vi "Modify Test Data.vi"(11 "Field Values in":T1={"cpu_temp"=48.25, "error_code"=-9003, "cpu_load"=8, "cpu_type"="Ryzen 5 2600", "cpu_busy?"=FALSE}) -> (2 "Variant":variant, 3 "Field Values out":T1={"cpu_temp"=48.25, "error_code"=-9003, "cpu_load"=8, "cpu_type"="Ryzen 5 2600", "cpu_busy?"=FALSE})   [LabVIEW 2020, in "InfluxDB v2 Client.lvlib"]
doc: "Modifies the test data with random values"
uses:
  InfluxDB v2 Client.lvlib
  Field Values.ctl
  <vilib>/numeric/Random Number (Range) U64.vi
  <vilib>/numeric/Random Number (Range) I64.vi
  <vilib>/numeric/Random Number (Range) DBL.vi
  <vilib>/numeric/sub_Random U32.vi
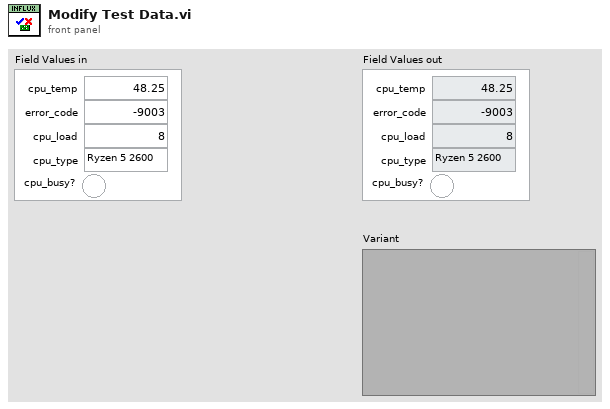
[diagram p1: front panel]
types:
  T1 = typedef "InfluxDB v2 Client.lvlib/Field Values.ctl" = cluster{"cpu_temp":dbl, "error_code":i64, "cpu_load":u64, "cpu_type":string, "cpu_busy?":bool}
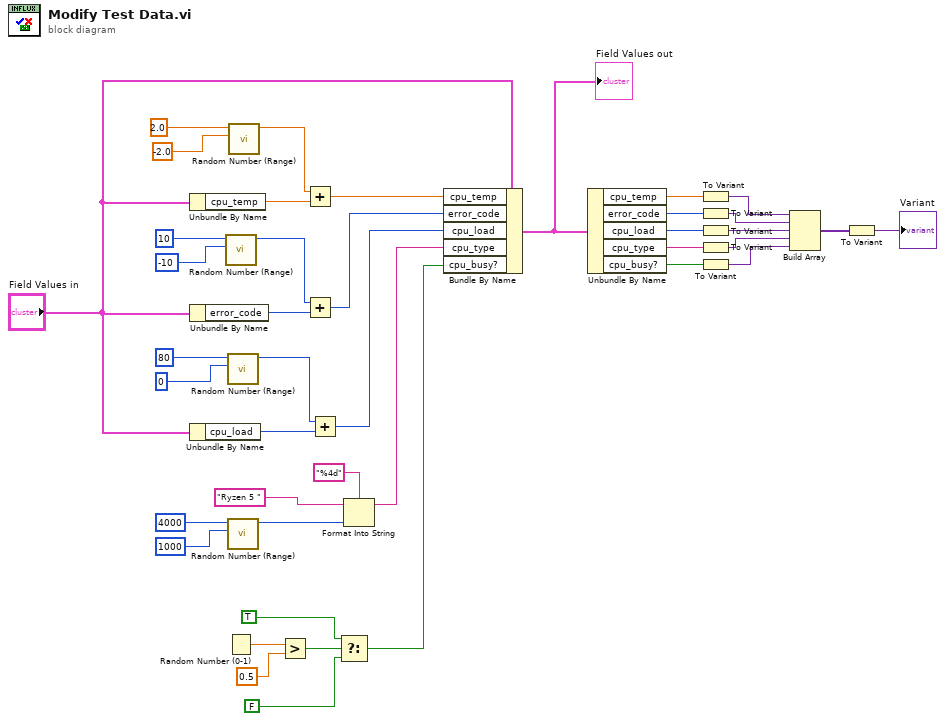
[diagram p0: block diagram]
diagram:
  n1 = Unbundle By Name("Field Values in") -> ("cpu_temp"=w39:dbl)
  n2 = Unbundle By Name("Field Values in") -> ("error_code"=w35:i64)
  n3 = Unbundle By Name("Field Values in") -> ("cpu_load"=w32:u64)
  n4 = call-poly <vilib>:"Random Number (Range).vi"("lower bound (-100)"=i64 -10 ("lower bound (0)"), "upper bound (100)"=i64 10) -> ("number"=w34:i64)  [unwired: 9 in]
  n5 = Random Number (0-1)() -> (number: 0 to 1=w24:dbl)
  n6 = call-poly <vilib>:"Random Number (Range).vi"("lower bound (0)"=u64 0, "upper bound (100)"=u64 80) -> ("number"=w33:u64)  [unwired: 9 in]
  n7 = call-poly <vilib>:"Random Number (Range).vi"("lower bound (0)"=u64 1000, "upper bound (100)"=u64 4000) -> ("number"=w26:u64)  [unwired: 9 in]
  n8 = call-poly <vilib>:"Random Number (Range).vi"("lower bound (0)"=-2.0, "upper bound (100)"=2.0) -> ("number"=w38:dbl)  [unwired: 9 in]
  n9 = Greater?(x=w24, y=0.5) -> (0:w22:bool)
  n10 = Add(x=w38, y=w39) -> (x+y=w18:dbl)
  n11 = Add(x=w34, y=w35) -> (x+y=w17:i64)
  n12 = Add(x=w33, y=w32) -> (x+y=w16:u64)
  n13 = Select(t=TRUE, s=w22, f=FALSE) -> (s? t:f=w14:bool)
  n14 = Format Into String(format string="%4d", initial string="Ryzen 5 ", w26) -> (resulting string=w15:string)  [unwired: 1 in, 1 out]
  n15 = Bundle By Name(cluster="Field Values in", "cpu_temp"=w18, "error_code"=w17, "cpu_load"=w16, "cpu_type"=w15, "cpu_busy?"=w14) -> (w13:T1)
  "Field Values out" <- w13
  n16 = Unbundle By Name(w13) -> ("cpu_temp"=w12:dbl, "error_code"=w11:i64, "cpu_load"=w10:u64, "cpu_type"=w9:string, "cpu_busy?"=w8:bool)
  n17 = To Variant(anything=w12) -> (Variant=w4:variant)
  n18 = To Variant(anything=w11) -> (Variant=w6:variant)
  n19 = To Variant(anything=w10) -> (Variant=w7:variant)
  n20 = To Variant(anything=w9) -> (Variant=w5:variant)
  n21 = To Variant(anything=w8) -> (Variant=w3:variant)
  n22 = Build Array(w4, w6, w7, w5, w3) -> (w2:variant[])
  n23 = To Variant(anything=w2) -> (Variant=→"Variant":variant)
